vi "Image.Load, Zoom and Center.vi"(6 "Center":bool=TRUE, 8 "error in (no error)":errorcluster, 9 "Zoom Factor":dbl, 10 "2D Pict Ref":refnum<vi>, 11 "File":path) -> (0 "error out":errorcluster, 3 "2D Pict":picture)   [LabVIEW 2018]
uses:
  <vilib>/KATE/Graphics/Graphic Utils.lvlib
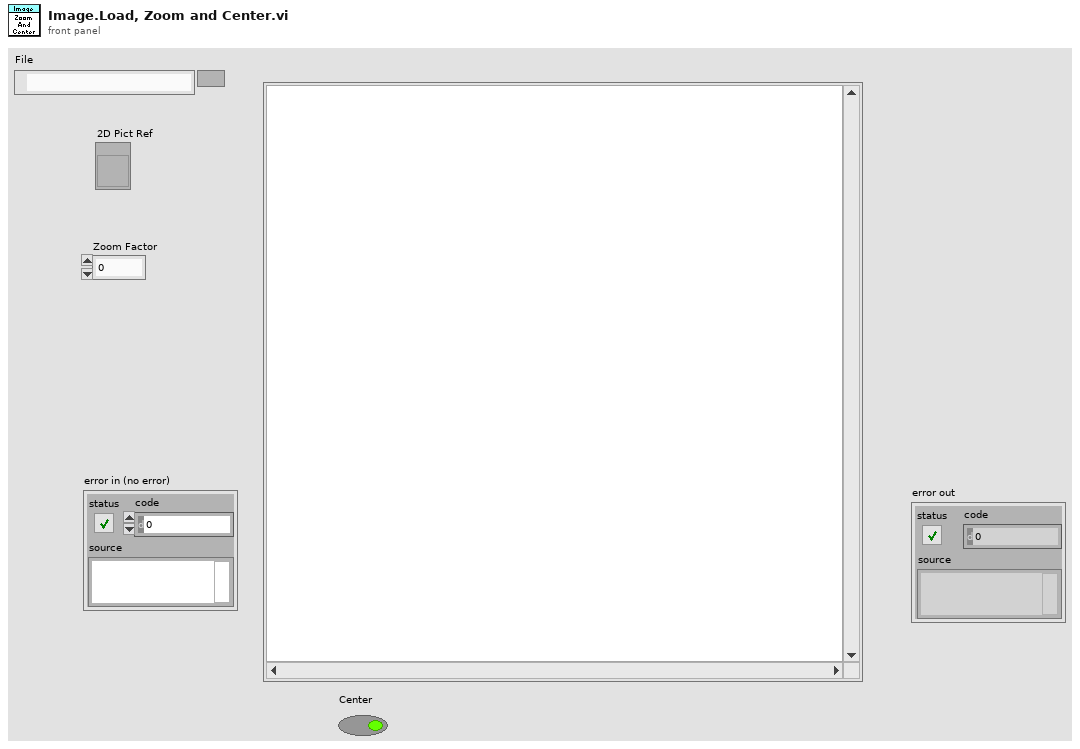
[diagram p1: front panel]
types:
  T1 = typedef "imagedata.ctl" = cluster{"image type":i32, "image depth":i32, "image":u8[], "mask":u8[], "colors":u32[], "Rectangle":cluster{"left":i16, "top":i16, "right":i16, "bottom":i16}}
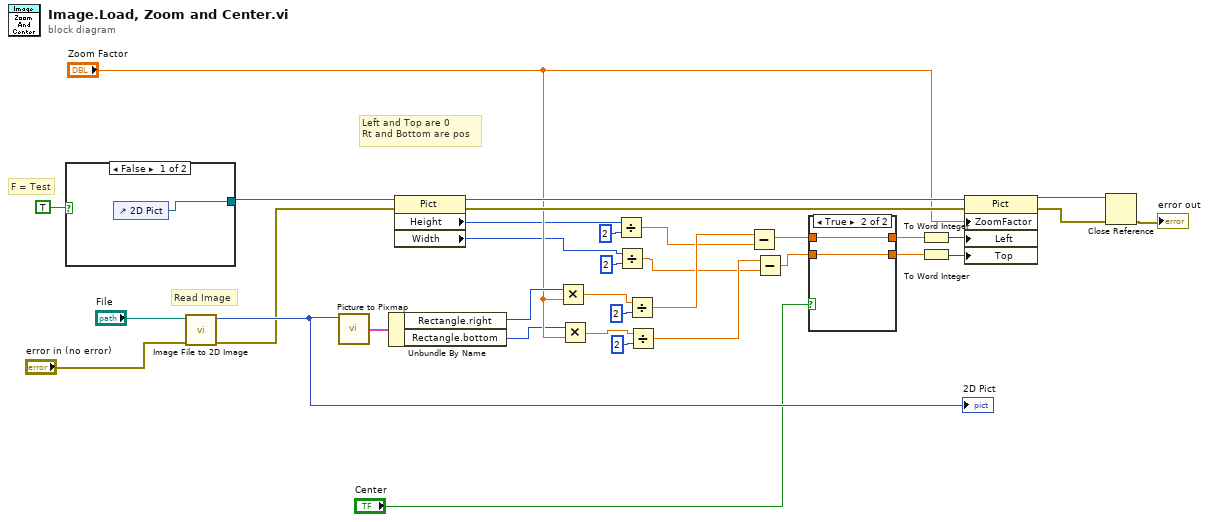
[diagram p0: block diagram]
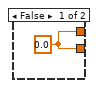
[diagram p2: hidden frame]
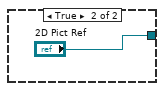
[diagram p3: hidden frame]
diagram:
  # "F = Test"
  # "Left and Top are 0\nRt and Bottom are pos"
  # "Read Image"
  n1 = case shown="False" TRUE {
    tunnel: [w35 "2D Pict Ref"] -> w31
    frame False {
      n2 = control-ref of="2D Pict"() -> (w35:refnum<vi>)
    }
    frame True {
    }
  }
  n3 = call <vilib>:"Image File to 2D Image.vi"("error in"="error in (no error)", "Path"="File") -> ("error out"=w26:errorcluster, "2D Picture"=w28:picture)  [unwired: 8 in]
  "2D Pict" <- w28
  n4 = call <vilib>:"Picture to Pixmap.vi"("picture"=w28) -> ("image data"=w32:T1)  [unwired: 9 in, 1 out]
  n5 = Unbundle By Name(w32) -> ("Rectangle.right"=w22:i16, "Rectangle.bottom"=w20:i16)
  n6 = property on="Property Node" class="Pict"(reference=w31, error in=w26) -> (reference out=w30:refnum<vi>, error out=w27:errorcluster, "Height"=w17:u32, "Width"=w14:u32)
  n7 = Multiply(x=w22, y="Zoom Factor") -> (x*y=w11:dbl)
  n8 = Multiply(x=w20, y="Zoom Factor") -> (x*y=w10:dbl)
  n9 = Divide(x=w17, y=u32 2) -> (x/y=w7:dbl)
  n10 = Divide(x=w14, y=u32 2) -> (x/y=w6:dbl)
  n11 = Divide(x=w11, y=u32 2) -> (x/y=w9:dbl)
  n12 = Divide(x=w10, y=u32 2) -> (x/y=w8:dbl)
  n13 = Subtract(x=w9, y=w7) -> (x-y=w2:dbl)
  n14 = Subtract(x=w8, y=w6) -> (x-y=w1:dbl)
  n15 = case shown="True" "Center" {
    tunnel: [w37 w39] -> w4
    tunnel: [w37 w38] -> w3
    tunnel: w2 -> [_ w39]
    tunnel: w1 -> [_ w38]
    frame False {
      w37 = 0.0
    }
    frame True {
    }
  }
  n16 = To Word Integer(number=w4) -> (16bit integer=w19:i16)
  n17 = To Word Integer(number=w3) -> (16bit integer=w18:i16)
  n18 = property on="Property Node" class="Pict"(reference=w30, error in=w27, "ZoomFactor"="Zoom Factor", "Left"=w19, "Top"=w18) -> (reference out=w25:refnum<vi>, error out=w24:errorcluster)
  n19 = Close Reference(reference=w25, error in (no error)=w24) -> (error out=→"error out":errorcluster)
